vi "UART Timeout.vi"(8 "error in (no error)":errorcluster, 11 "Timeout (s)":i32=3) -> (0 "error out":errorcluster)   [LabVIEW 2011]
uses:
  Libraries/uart_library.dll
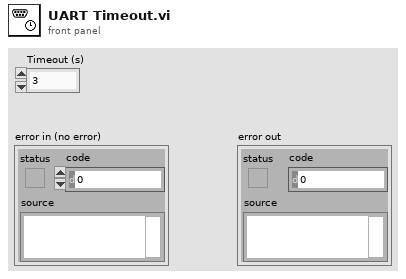
[diagram p1: front panel]
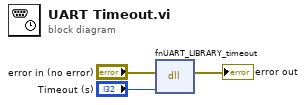
[diagram p0: block diagram]
diagram:
  n1 = dll-call lib="E:/users/tba/work_project/FW102/trunk/LabVIEW/Libraries/uart_library.dll" fn="fnUART_LIBRARY_timeout"(error in="error in (no error)", "Timeout"="Timeout (s)") -> (error out=→"error out":errorcluster)  [unwired: 4 in, 1 out]
